vi "Query Measurement.vi"(8 "error in (no error)":errorcluster, 10 "States":dbl[](array[numeric]), 11 "LCR Meter in":refnum<class "LCR Meter.lvclass">) -> (0 "error out":errorcluster, 1 "Secondary results":dbl[](array[numeric]), 2 "Capacitances (fF)":dbl[](array[numeric]), 3 "LCR Meter out":refnum<class "LCR Meter.lvclass">)   [LabVIEW 2020, in "LCR Meter.lvclass"]
uses:
  LCR Meter.lvclass
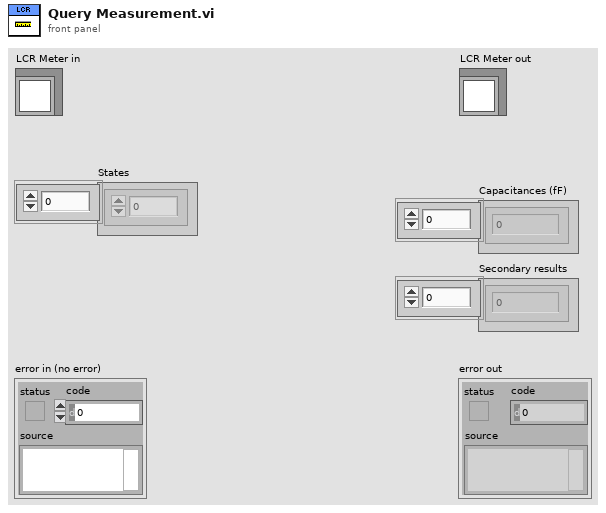
[diagram p1: front panel]
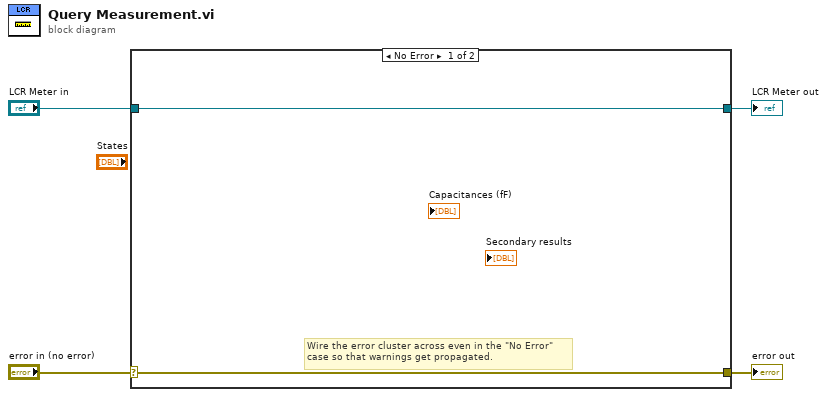
[diagram p0: block diagram]
diagram:
  n1 = case shown="No Error" "error in (no error)" {
    selector: "error in (no error)" -> [w5 w8]
    tunnel: [w5 w8] -> w3
    tunnel: [w6 w7] -> w1
    tunnel: "LCR Meter in" -> [w6 w7]
    frame No Error {
      # "Wire the error cluster across even in the \"No Error\"\ncase so that warnings get propagated."
    }
    frame Error {
    }
  }
  "error out" <- w3
  "LCR Meter out" <- w1
